vi "Get Faults.vi"(0 "object in":refnum<class "HPS-17000-PowerModule.lvclass">, 11 "Error In":errorcluster) -> (4 "object out":refnum<class "HPS-17000-PowerModule.lvclass">, 6 "active faults":string[](array[string]), 8 "fault":bool, 15 "Error Out":errorcluster)   [LabVIEW 2023, in "HPS-17000-PowerModule.lvlib" / "HPS-17000-PowerModule.lvclass"]
uses:
  HPS-17000-PowerModule.lvclass
  <instrlib>/HPS-17000/Internal/Get Faults Multi.vi
  <instrlib>/HPS-17000/HPS-17000.lvclass
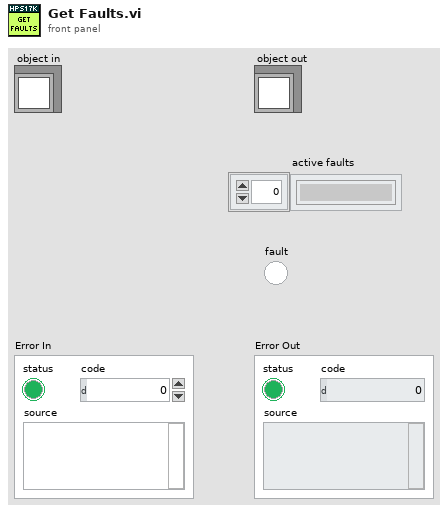
[diagram p1: front panel]
types:
  T1 = typedef "HPS-17000-PowerModule.lvlib/HPS-17000-PowerModule.lvclass/ObjectAttributes.ctl" = cluster{"HPS17000 IP Addresses":string[], "HPS Topology":enum16{"SINGLE", "MULTI"}, "GM ID":string, "TSN NIC IP Address":string, "HPS17000 Refs":refnum<class "HPS-17000.lvclass">[], "Stream Queues":refnum<queue>[], "connected":bool, "reserved":bool, "events":T2, "nibatterycycler_grpc_Setpoint":T3, "last timestamp":i64, "setpoint stream config":T4, "mode":T5, "range":T6}
  T2 = typedef "HPS-17000.lvclass/Multi-Cycler Events.ctl" = cluster{"heartbeats events":refnum<user-event>[], "faults events":refnum<user-event>[], "network sync event":refnum<user-event>[], "setpoint status event":refnum<user-event>[]}
  T3 = typedef "NI_BC_client.lvlib/nibatterycycler_grpc_Setpoint.ctl" = cluster{"voltage":sgl, "current":sgl, "min_power":sgl, "max_power":sgl, "resistance":sgl}
  T4 = typedef "Cycler.lvclass/Setpoint Stream Basic Config.ctl" = cluster{"local address":string, "receiver port":u16}
  T5 = typedef "HPS-17000-PowerModule.lvlib/HPS-17000-PowerModule.lvclass/Mode.ctl" = u16
  T6 = typedef "PowerModuleInterface.lvlibp/PowerModuleInterface.lvclass/Range.ctl" = cluster{"Current Max (A)":dbl, "Current Min (A)":dbl, "Voltage Max (V)":dbl, "Voltage Min (V)":dbl}
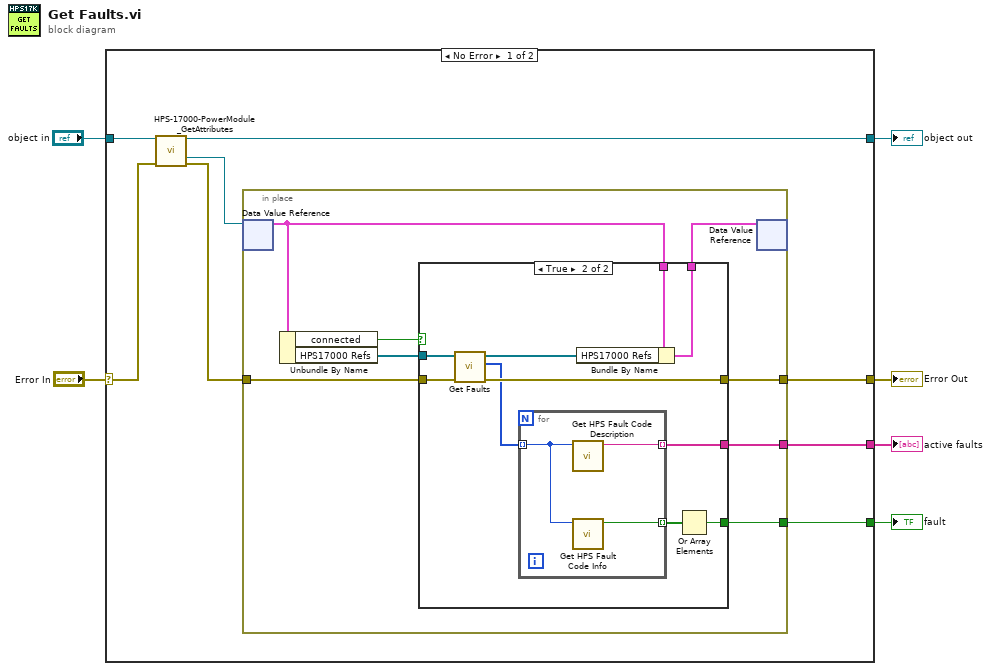
[diagram p0: block diagram]
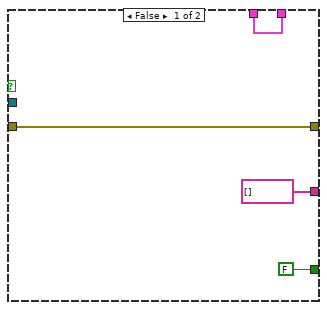
[diagram p2: hidden frame]
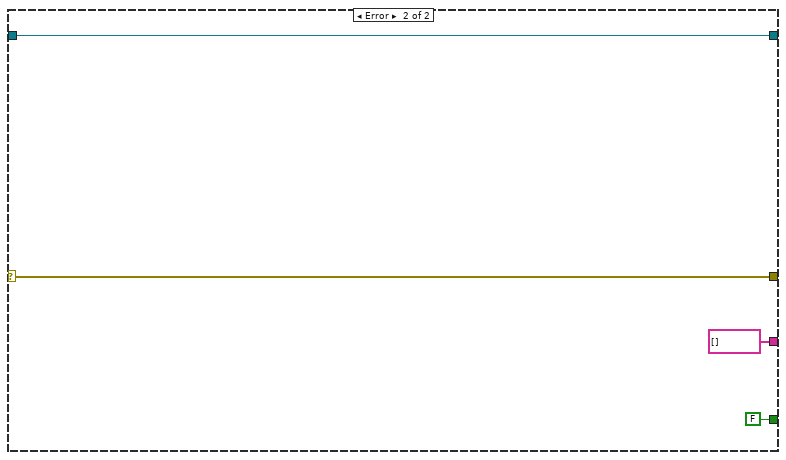
[diagram p3: hidden frame]
diagram:
  n1 = case shown="No Error" "Error In" {
    selector: "Error In" -> [w13 w42]
    tunnel: "object in" -> [w14 w43]
    tunnel: [w9 w43] -> w5
    tunnel: [w10 w42] -> w3
    tunnel: [w8 FALSE] -> w2
    tunnel: [w7 string[] []] -> w1
    frame No Error {
      n2 = call "HPS-17000-PowerModule_GetAttributes.vi"("reference in"=w14, "Error In"=w13) -> ("reference out"=w9:refnum<class "HPS-17000-PowerModule.lvclass">, "DataRef"=w12:refnum<data-value>, "Error Out"=w11:errorcluster)  [unwired: 10 in, 1 out]
      n3 = in-place {
        in-place-border: w11 -> [w20]
        in-place-border: [w19] -> w10
        in-place-border: [w16] -> w8
        in-place-border: [w15] -> w7
        n4 = in-place-dvr #1(w12) -> (w21:T1)  [unwired: 1 out]
        n5 = Unbundle By Name(w21) -> ("connected"=w17:bool, "HPS17000 Refs"=w18:refnum<class "HPS-17000.lvclass">[])
        n6 = case shown="True" w17 {
          tunnel: [w26 w36] -> w22
          tunnel: w21 -> [w26 w35]
          tunnel: w20 -> [w25 w34]
          tunnel: [w25 w32] -> w19
          tunnel: w18 -> [_ w33]
          tunnel: [FALSE w28] -> w16
          tunnel: [string[] [] w27] -> w15
          frame False {
          }
          frame True {
            n7 = call-poly <instrlib>:"Get Faults.vi"("error in"=w34, "cycler refs in"=w33) -> ("error out"=w32:errorcluster, "faults"=w30:u64[], "cycler refs out"=w31:refnum<class "HPS-17000.lvclass">[])  [unwired: 7 in]
            n8 = for {
              tunnel: w30 -> [w39] mode=indexing
              tunnel: [w38] -> w29 mode=indexing
              tunnel: [w37] -> w27 mode=indexing
              n9 = call "Get HPS Fault Code Description.vi"("fault code"=w39) -> ("fault description"=w37:string)  [unwired: 10 in]
              n10 = call "Get HPS Fault Code Info.vi"("fault code"=w39) -> ("is fault?"=w38:bool)  [unwired: 8 in, 2 out]
            }
            n11 = Bundle By Name(cluster=w35, "HPS17000 Refs"=w31) -> (w36:T1)
            n12 = Or Array Elements(Boolean array=w29) -> (logical OR=w28:bool)
          }
        }
        n13 = in-place-dvr #1(w22) -> ()  [unwired: 2 out]
      }
    }
    frame Error {
    }
  }
  "Error Out" <- w3
  "object out" <- w5
  "active faults" <- w1
  "fault" <- w2
